vi "Define.vi"(11 "Definition":T1={"Type"={"Name"="", "Nullable"=FALSE, "Default NULL"=FALSE}, "Attributes"={"Primary Key"=FALSE, "Unique"=FALSE, "Foreign Key"=FALSE, "Auto Increment"=FALSE}, "String"={"Default"="", "Length"=255}}) -> (3 "String out":refnum<class "String.lvclass">)   [LabVIEW 2020, in "Conditum.lvlib" / "Columns.lvlib" / "String.lvclass"]
uses:
  String.lvclass
  Type/Type.lvclass
  LabVIEW Type.ctl
  Conditum.lvlib
  C:/dev/lv/illuminated-g/lv-conditum/Conditum/Columns/Type/Type.lvclass
  Type/Definition.ctl
  Definition.ctl
  String Definition.ctl
  Attributes.ctl
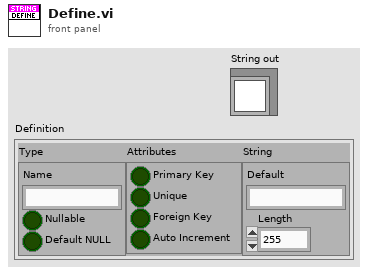
[diagram p1: front panel]
types:
  T1 = typedef "Conditum.lvlib/Columns.lvlib/String.lvclass/String Definition.ctl" = cluster{"Type":T2, "Attributes":T3, "String":T4}
  T2 = typedef "Conditum.lvlib/Columns.lvlib/Type.lvclass/Definition.ctl" = cluster{"Name":string, "Nullable":bool, "Default NULL":bool}
  T3 = typedef "Conditum.lvlib/Attributes.ctl" = cluster{"Primary Key":bool, "Unique":bool, "Foreign Key":bool, "Auto Increment":bool}
  T4 = typedef "Conditum.lvlib/Columns.lvlib/String.lvclass/Definition.ctl" = cluster{"Default":string, "Length":i32}
  T5 = typedef "Conditum.lvlib/LabVIEW Type.ctl" = enum16{"None", "ID", "Boolean", "Integer", "Double", "Timestamp", "String", "Text", "Entity"}
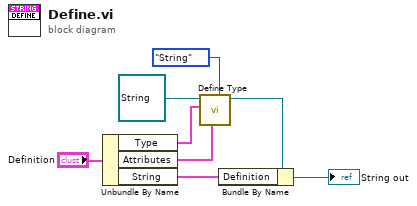
[diagram p0: block diagram]
diagram:
  n1 = Unbundle By Name("Definition") -> ("Type"=w6:T2, "Attributes"=w2:T3, "String"=w5:T4)
  n2 = call "Define Type.vi"("Type"=LabVIEW_Type."String", "Attributes"=w2, "Definition"=w6, "Type in"=refnum<class "String.lvclass"> refnum ("String out")) -> ("Type out"=w4:refnum<class "String.lvclass">)  [unwired: 7 in]
  n3 = Bundle By Name(cluster=w4, "Definition"=w5) -> (→"String out":refnum<class "String.lvclass">)
